vi "Self-Test.vi"(8 "error in (no error)":errorcluster, 11 "BH Druck PACE Series in":refnum<class "BH Druck PACE Series.lvclass">) -> (0 "error out":errorcluster, 1 "Self-Test Result Message":string, 2 "Self-Test Result Code":i32, 3 "BH Druck PACE Series out":refnum<class "BH Druck PACE Series.lvclass">)   [LabVIEW 2022 SP3, in "BH Druck PACE Series.lvclass"]
uses:
  BH Druck PACE Series.lvclass
  BH Druck PACE Series.lvclass/BH Druck PACE Series.ctl
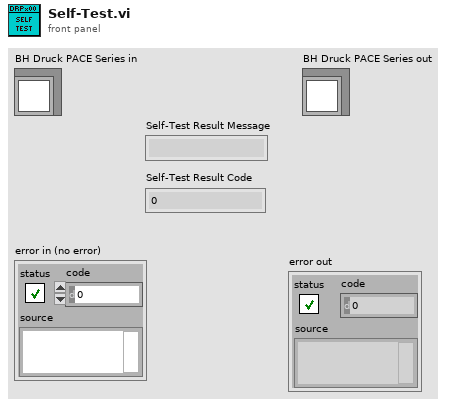
[diagram p1: front panel]
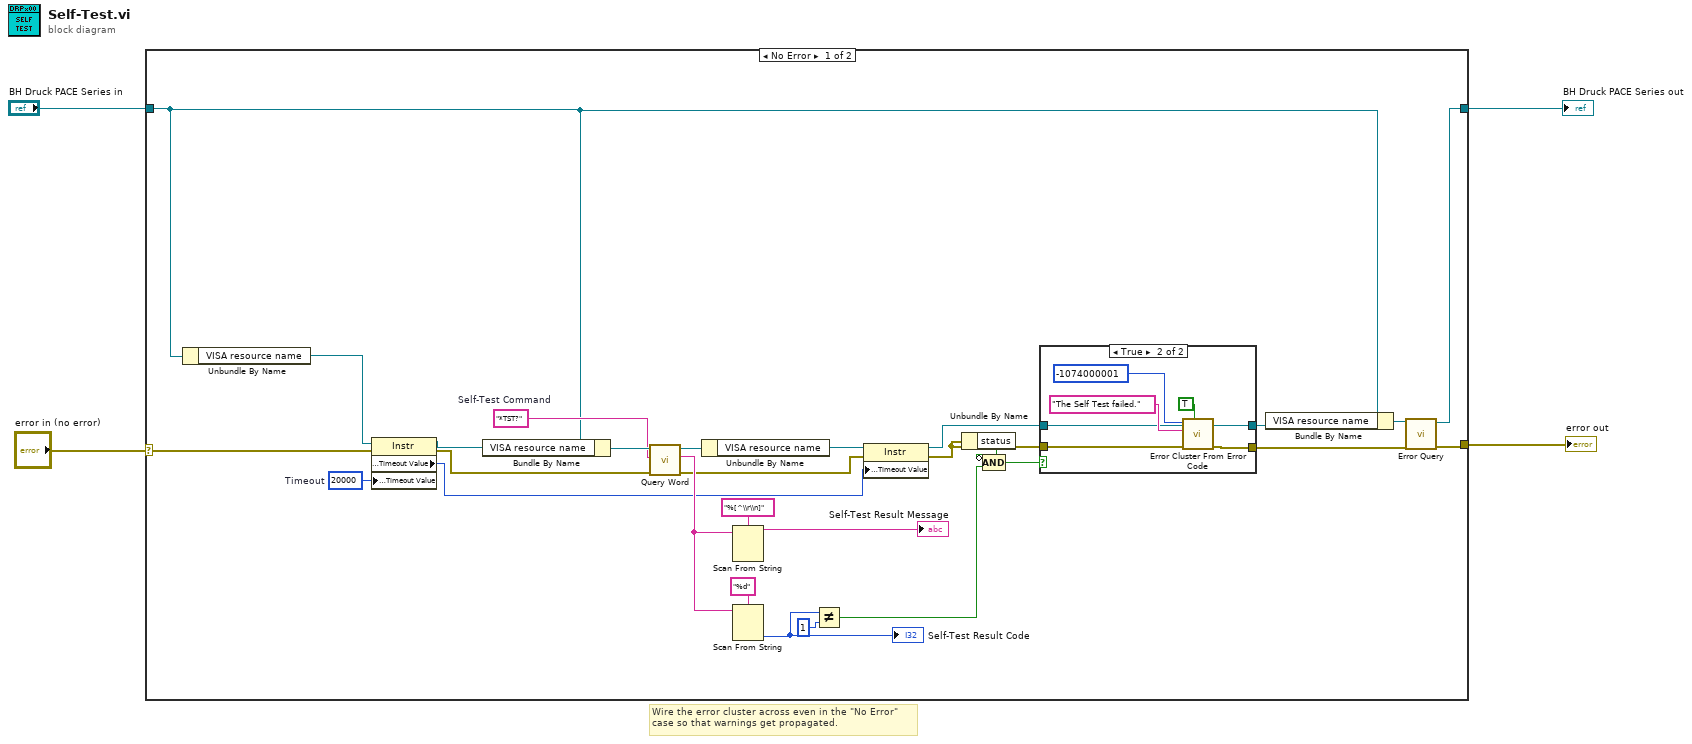
[diagram p0: block diagram]
diagram:
  # "Wire the error cluster across even in the \"No Error\"\ncase so that warnings get propagated."
  n1 = case shown="No Error" "error in (no error)" {
    selector: "error in (no error)" -> [w31 w42]
    tunnel: [w10 w42] -> w3
    tunnel: [w8 w41] -> w1
    tunnel: "BH Druck PACE Series in" -> [w13 w41]
    frame No Error {
      w26 = "*TST?"  # Self-Test Command
      w32 = u32 20000  # Timeout
      n2 = Unbundle By Name(w13) -> ("VISA resource name"=w30:refnum<visa-resource-name>)
      n3 = property on="Property Node" class="Instr"(reference=w30, error in=w31, "General Settings:Timeout Value"=w32) -> (reference out=w29:refnum<visa-resource-name>, error out=w27:errorcluster, "General Settings:Timeout Value"=w5:u32)
      n4 = Bundle By Name(cluster=w13, "VISA resource name"=w29) -> (w28:refnum<class "BH Druck PACE Series.lvclass">)
      n5 = call-dynamic "Query Word.vi"("error in (no error)"=w27, "Query String"=w26, "BH Druck PACE Series in"=w28) -> ("error out"=w14:errorcluster, "String Result"=w15:string, "BH Druck PACE Series out"=w7:refnum<class "BH Druck PACE Series.lvclass">)  [unwired: 6 in]
      n6 = Unbundle By Name(w7) -> ("VISA resource name"=w6:refnum<visa-resource-name>)
      n7 = Scan From String(format string="%[^\\r\\n]" ("Format String"), input string=w15) -> (output 1=→"Self-Test Result Message":string)  [unwired: 3 in, 3 out]
      n8 = Scan From String(format string="%d", input string=w15) -> (output 1=w20:i32)  [unwired: 3 in, 3 out]
      "Self-Test Result Code" <- w20
      n9 = Not Equal?(x=w20, y=1) -> (x != y?=w22:bool)
      n10 = property on="Property Node" class="Instr"(reference=w6, error in=w14, "General Settings:Timeout Value"=w5) -> (reference out=w16:refnum<visa-resource-name>, error out=w18:errorcluster)
      n11 = Unbundle By Name(w18) -> ("status"=w21:bool)
      n12 = Compound Arithmetic op=AND(invert w21, w22) -> (w17:bool)
      n13 = case shown="True" w17 {
        tunnel: w18 -> [w34 w35]
        tunnel: [w34 w37] -> w11
        tunnel: w16 -> [w33 w36]
        tunnel: [w33 w36] -> w12
        frame False {
        }
        frame True {
          n14 = call <vilib>:"Error Cluster From Error Code.vi"("show call chain? (False)"=TRUE, "error in (no error)"=w35, "error message (\"\")"="The Self Test failed." ("Source (VI Name)"), "error code (0)"=-1074000001 ("Code")) -> ("error out"=w37:errorcluster)  [unwired: 5 in]
        }
      }
      n15 = Bundle By Name(cluster=w13, "VISA resource name"=w12) -> (w9:refnum<class "BH Druck PACE Series.lvclass">)
      n16 = call-dynamic "Error Query.vi"("error in (no error)"=w11, "BH Druck PACE Series in"=w9) -> ("error out"=w10:errorcluster, "BH Druck PACE Series out"=w8:refnum<class "BH Druck PACE Series.lvclass">)  [unwired: 8 in]
    }
    frame Error {
    }
  }
  "error out" <- w3
  "BH Druck PACE Series out" <- w1
